vi "fgv_5413_config.vi"(7 "cmd":T2, 11 "config":T1={"visa"="", "DC Offset"=0.0, "Digital Filter"=FALSE, "Analog Filter"=FALSE, "Tones"=[{"Frequency"=1000000.0, "Amplitude"=0.5, "Phase"=0.0}, {"Frequency"=1100000.0, "Amplitude"=0.5, "Phase"=0.0}], "Sampling Info"={"Frequency"=20000000.0, "Number of Samples"=10000.0}, "Clock Mode"=1, "Sample Rate (S/s)"=20000000.0, "Gain"=0.0, "Sample Clock Source"="OnboardClock"} {"Sample Rate (S/s)" format="%.2p"; "Clock Mode" items=["Hi Resolution Sampling", "Divide Down Sampling", "Automatic"]; "Sampling Info"."Frequency" format="%.2p"; "Tones"."Phase" format="%.2p"; "Tones"."Amplitude" format="%.2p"; "Tones"."Frequency" format="%.2p"}) -> (3 "config 2":T1={"visa"="", "DC Offset"=0.0, "Digital Filter"=FALSE, "Analog Filter"=FALSE, "Tones"=[{"Frequency"=1000000.0, "Amplitude"=0.5, "Phase"=0.0}, {"Frequency"=1100000.0, "Amplitude"=0.5, "Phase"=0.0}], "Sampling Info"={"Frequency"=20000000.0, "Number of Samples"=10000.0}, "Clock Mode"=1, "Sample Rate (S/s)"=20000000.0, "Gain"=0.0, "Sample Clock Source"="OnboardClock"} {"Sample Rate (S/s)" format="%.2p"; "Clock Mode" items=["Hi Resolution Sampling", "Divide Down Sampling", "Automatic"]; "Sampling Info"."Frequency" format="%.2p"; "Tones"."Phase" format="%.2p"; "Tones"."Amplitude" format="%.2p"; "Tones"."Frequency" format="%.2p"})   [LabVIEW 2021]
uses:
  ctrl/rw.ctl
  ctrl/PXIe-5413_cfg.ctl
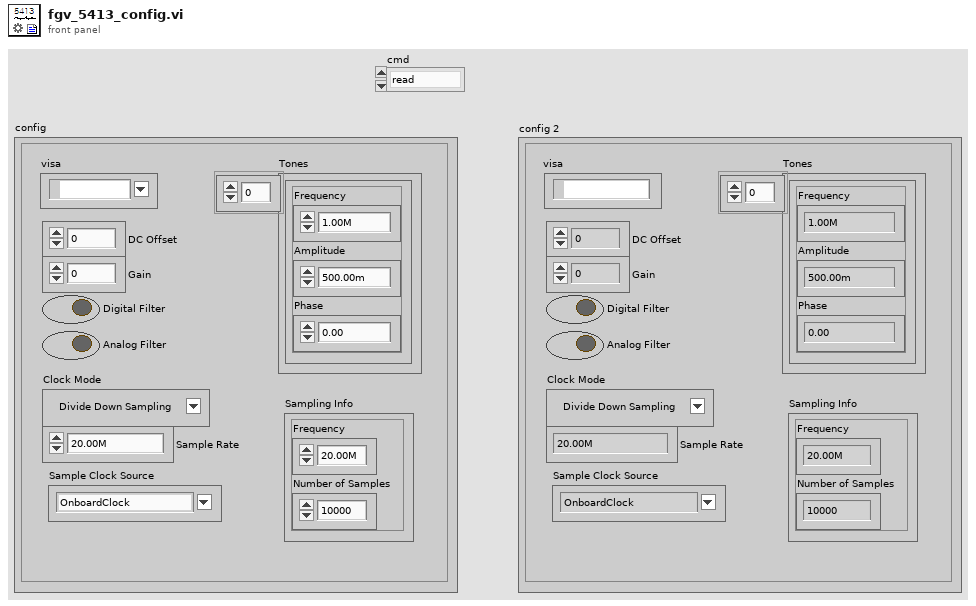
[diagram p1: front panel]
types:
  T1 = typedef "PXIe-5413_cfg.ctl" = cluster{"visa":refnum<k15>, "DC Offset":dbl, "Digital Filter":bool, "Analog Filter":bool, "Tones":cluster{"Frequency":dbl, "Amplitude":dbl, "Phase":dbl}[], "Sampling Info":cluster{"Frequency":dbl, "Number of Samples":dbl}, "Clock Mode":u32, "Sample Rate (S/s)":dbl, "Gain":dbl, "Sample Clock Source":string}
  T2 = typedef "rw.ctl" = enum16{"read", "write"}
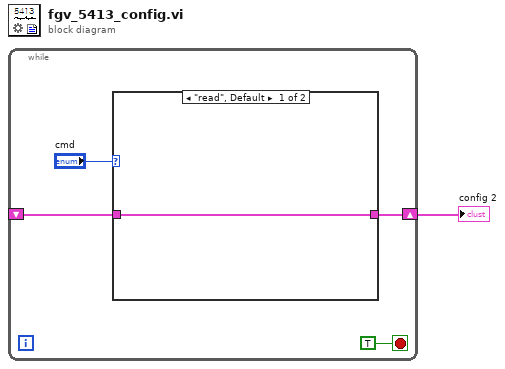
[diagram p0: block diagram]
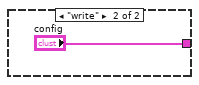
[diagram p2: hidden frame]
diagram:
  n1 = while {
    shift-right: [w3] -> w1
    shift-left: _ -> [w2]
    stop <- TRUE stop-if-true
    n2 = case shown="\"read\", Default" "cmd" {
      tunnel: [w6 "config"] -> w3
      tunnel: w2 -> [w6 _]
      frame "read", Default {
      }
      frame "write" {
      }
    }
  }
  "config 2" <- w1
